vi "Delimiter.vi"() -> ()   [LabVIEW 2017]
panel:
  in  "Delimiter":string=";"
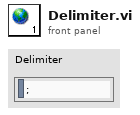
[diagram p1: front panel]
diagram:
